vi "FMSCount.vi"(4 "DIO Outtake":T1, 6 "Eval Period Out":dbl, 10 "Eval Period Intake":dbl(knob)=0.09675480749258313 scale=0.0..1.0, 11 "reset":bool) -> (1 "Total Outtook":dbl, 2 "Current Number":dbl, 3 "Total Intook":dbl)   [LabVIEW 2016]
uses:
  <vilib>/Rock Robotics/WPI/DigitalInput/WPI_DigitalInputDevRef.ctl
  <vilib>/Rock Robotics/SystemInterfaces/DIO/FPGA_DIOChannel.ctl
  <vilib>/Platform/TimedLoop/XDataNode/timing_clust.ctl
  <vilib>/Platform/TimedLoop/XDataNode/nitl_modes.ctl
  <vilib>/Platform/TimedLoop/XDataNode/wakeup.ctl
  <vilib>/platform/TimedLoop/XDataNode/XDataNode.xnode
  <vilib>/Platform/TimedLoop/XDataNode/XDNodeRunTimeDep.lvlib
panel:
  in  "DIO Intake":T3
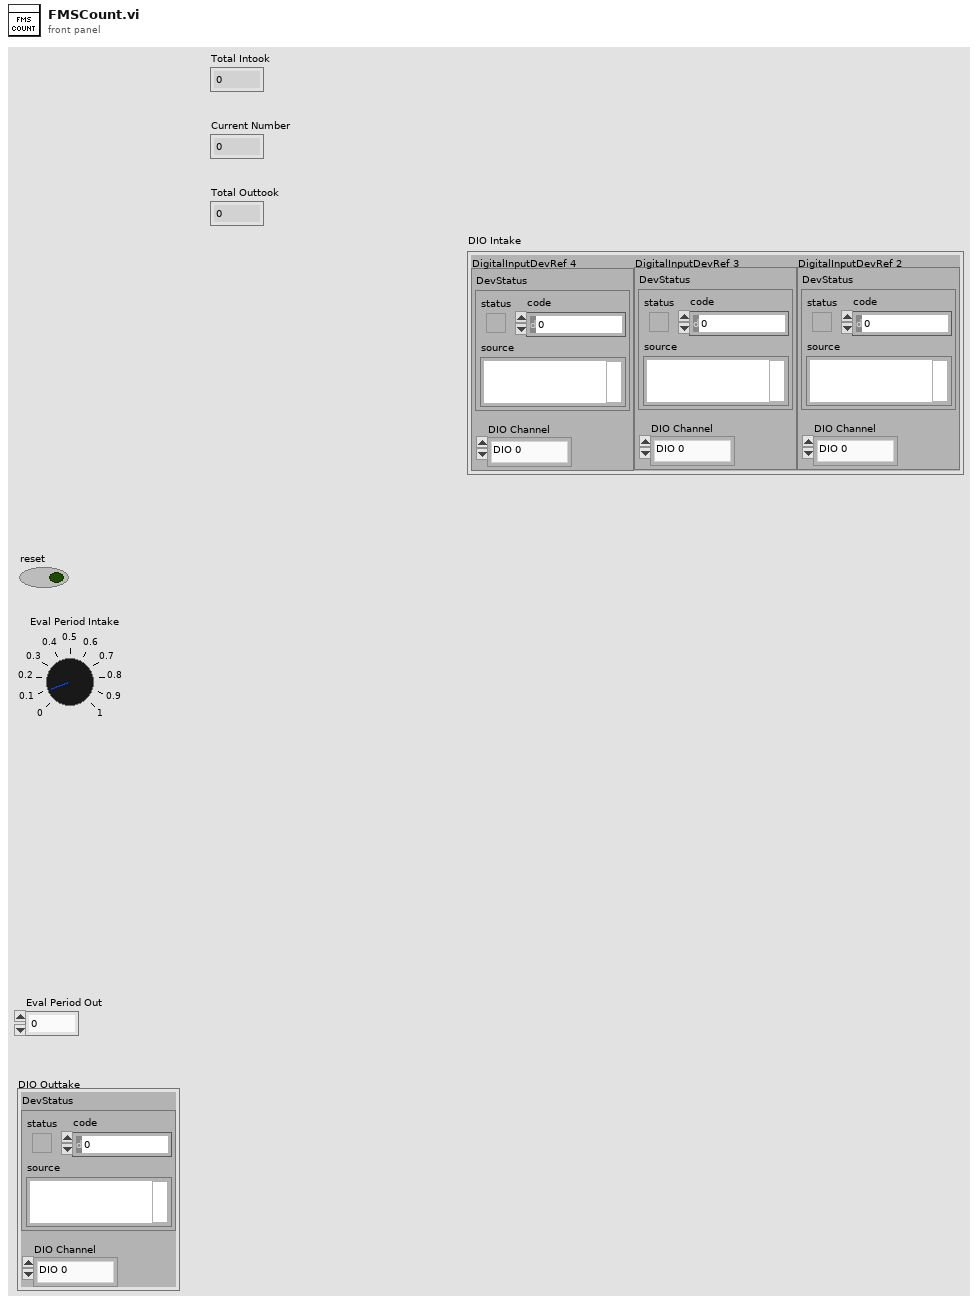
[diagram p1: front panel]
types:
  T1 = typedef "WPI_DigitalInputDevRef.ctl" = cluster{"DevStatus":errorcluster, "DIO Channel":T2}
  T2 = typedef "FPGA_DIOChannel.ctl" = enum8{"DIO 0", "DIO 1", "DIO 2", "DIO 3", "DIO 4", "DIO 5", "DIO 6", "DIO 7", "DIO 8", "DIO 9", "DIO MXP 0", "DIO MXP 1", "DIO MXP 2", "DIO MXP 3", "DIO MXP 4", "DIO MXP 5", "DIO MXP 6", "DIO MXP 7", "DIO MXP 8", "DIO MXP 9", "DIO MXP 10", "DIO MXP 11", "DIO MXP 12", "DIO MXP 13", "DIO MXP 14", "DIO MXP 15", "SPI Port CS1", "SPI Port CS2", "SPI Port CS3", "SPI Port MISO", "SPI Port MOSI", "Invalid"}
  T3 = cluster{"DigitalInputDevRef 4":T1, "DigitalInputDevRef 3":T1, "DigitalInputDevRef 2":T1}
  T4 = typedef "XDNodeRunTimeDep.lvlib/timing_clust.ctl" = cluster{"Expected End [f-1]":u64, "Actual End [f-1]":u64, "Finished Late? [f-1]":bool, "Expected End [i-1]":u64, "Actual End [i-1]":u64, "Finished Late? [i-1]":bool, "Expected Start [i]":u64, "Actual Start [i]":u64, "Expected Start [f]":u64, "Actual Start [f]":u64, "Source Name":string, "Structure Name":string, "Period":i64, "Deadline":i64, "Offset":i64, "Start":i64, "Priority":i32, "Timeout":i32, "Mode":T5, "Wakeup Reason":T6, "Error":errorcluster, "Source Type":string, "Secondary Source Type":string, "Global End Time":u64, "Global Start Time":u64, "Frame Duration":u64, "Iteration Duration":u64, "Assigned CPU":i32, "I/O Scan Engine Mode":u32}
  T5 = typedef "XDNodeRunTimeDep.lvlib/nitl_modes.ctl" = enum32{"No Change", "Process missed periods, maintain original phase", "Discard missed periods, maintain original phase", "Process missed periods, ignore original phase", "Discard missed periods, ignore original phase"}
  T6 = typedef "XDNodeRunTimeDep.lvlib/wakeup.ctl" = enum32{"Normal", "Aborted", "Asynchronous wakeup", "Timing source error", "Timed loop error", "Timeout"}
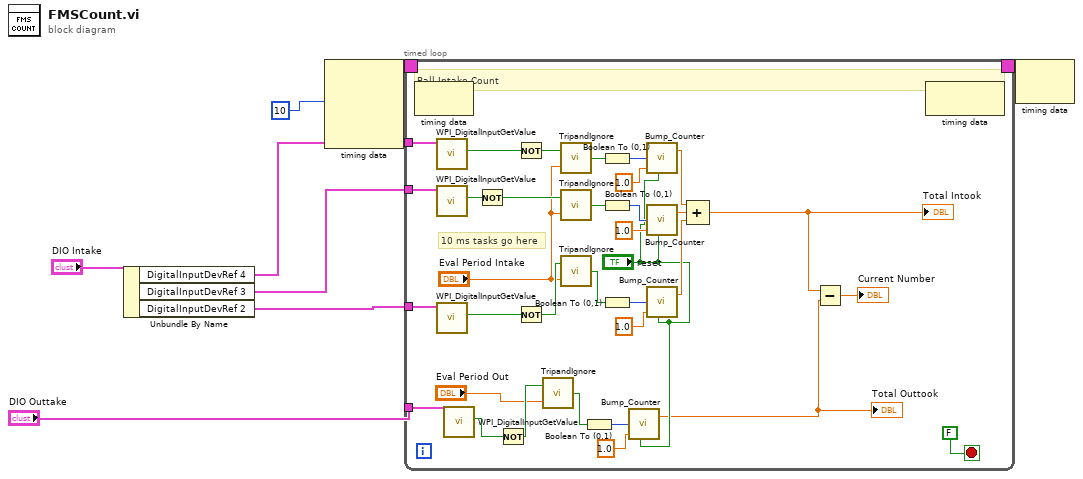
[diagram p0: block diagram]
diagram:
  n1 = Unbundle By Name("DIO Intake") -> ("DigitalInputDevRef 4"=w6:T1, "DigitalInputDevRef 3"=w5:T1, "DigitalInputDevRef 2"=w4:T1)
  n2 = node-c288(u32 10 ("milliseconds to wait")) -> (w3:T4)  [unwired: 3 in]
  n3 = timed-loop {
    tunnel: w6 -> [w41]
    tunnel: w5 -> [w40]
    tunnel: w4 -> [w39]
    tunnel: "DIO Outtake" -> [w19]
    timing: w3 -> [_]
    timing-out: [_] -> w2
    stop <- FALSE stop-if-true
    # "10 ms tasks go here"
    # "Ball Intake Count"
    n4 = node-c288() -> ()  [unwired: 1 in, 1 out]
    n5 = call <vilib>:"WPI_DigitalInputGetValue.vi"("DigitalInputDevRef"=w41) -> ("Value"=w38:bool)  [unwired: 8 in, 2 out]
    n6 = call <vilib>:"WPI_DigitalInputGetValue.vi"("DigitalInputDevRef"=w40) -> ("Value"=w37:bool)  [unwired: 8 in, 2 out]
    n7 = call <vilib>:"WPI_DigitalInputGetValue.vi"("DigitalInputDevRef"=w39) -> ("Value"=w36:bool)  [unwired: 8 in, 2 out]
    n8 = call <vilib>:"WPI_DigitalInputGetValue.vi"("DigitalInputDevRef"=w19) -> ("Value"=w15:bool)  [unwired: 8 in, 2 out]
    n9 = Not(x=w37) -> (.not. x?=w24:bool)
    n10 = Not(x=w15) -> (.not. x?=w14:bool)
    n11 = Not(x=w38) -> (.not. x?=w22:bool)
    n12 = Not(x=w36) -> (.not. x?=w26:bool)
    n13 = call "TripandIgnore.vi"("Eval Period (s)"="Eval Period Out", "Signal In"=w14) -> ("Tripped?"=w16:bool)
    n14 = call "TripandIgnore.vi"("Eval Period (s)"="Eval Period Intake", "Signal In"=w22) -> ("Tripped?"=w20:bool)
    n15 = call "TripandIgnore.vi"("Eval Period (s)"="Eval Period Intake", "Signal In"=w24) -> ("Tripped?"=w23:bool)
    n16 = call "TripandIgnore.vi"("Eval Period (s)"="Eval Period Intake", "Signal In"=w26) -> ("Tripped?"=w25:bool)
    n17 = Boolean To (0,1)(Boolean=w16) -> (0, 1=w18:i16)
    n18 = Boolean To (0,1)(Boolean=w20) -> (0, 1=w33:i16)
    n19 = Boolean To (0,1)(Boolean=w23) -> (0, 1=w35:i16)
    n20 = Boolean To (0,1)(Boolean=w25) -> (0, 1=w34:i16)
    n21 = call <userlib>:"Bump_Counter.vi"("cntrl"=w18, "quanta"=1.0, "reset"="reset") -> ("out"=w10:dbl)  [unwired: 3 in]
    "Total Outtook" <- w10
    n22 = call <userlib>:"Bump_Counter.vi"("cntrl"=w33, "quanta"=1.0, "reset"="reset") -> ("out"=w32:dbl)  [unwired: 3 in]
    n23 = call <userlib>:"Bump_Counter.vi"("cntrl"=w35, "quanta"=1.0, "reset"="reset") -> ("out"=w31:dbl)  [unwired: 3 in]
    n24 = call <userlib>:"Bump_Counter.vi"("cntrl"=w34, "quanta"=1.0, "reset"="reset") -> ("out"=w30:dbl)  [unwired: 3 in]
    n25 = Compound Arithmetic op=ADD(w32, w31, w30) -> (w11:dbl)
    "Total Intook" <- w11
    n26 = Subtract(x=w11, y=w10) -> (x-y=→"Current Number":dbl)
    n27 = node-c288() -> ()  [unwired: 1 in, 1 out]
  }
  n28 = node-c288(w2) -> ()  [unwired: 1 out]
